vi "Retrieve and Convert Data.vi"(8 "error in (no error)":errorcluster, 11 "Variant In":variant) -> (0 "error out":errorcluster, 2 "Info":T1, 3 "Variant Out":variant)   [LabVIEW 2019, in "Inset.lvclass"]
uses:
  Inset.lvclass
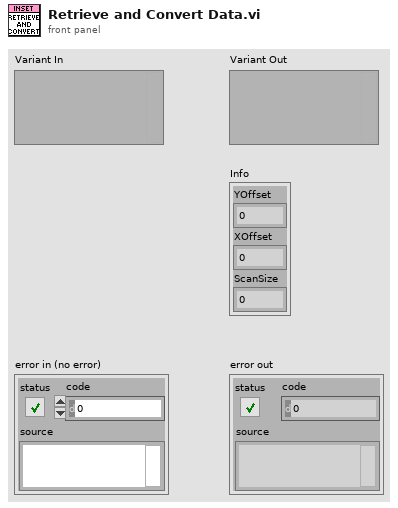
[diagram p1: front panel]
types:
  T1 = cluster{"YOffset":dbl, "XOffset":dbl, "ScanSize":dbl}
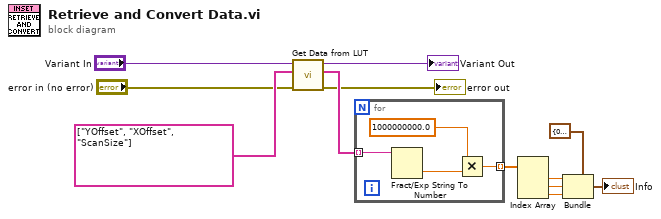
[diagram p0: block diagram]
diagram:
  n1 = call "Get Data from LUT.vi"("error in"="error in (no error)", "Keys"=string[] ["YOffset", "XOffset", "ScanSize"], "Variant In"="Variant In") -> ("error out"=→"error out":errorcluster, "Values"=w5:string[], "Variant Out"=→"Variant Out":variant)  [unwired: 6 in]
  n2 = for {
    tunnel: w5 -> [w16] mode=indexing
    tunnel: [w14] -> w12 mode=indexing
    n3 = Fract/Exp String To Number(string=w16) -> (number=w15:dbl)  [unwired: 3 in, 1 out]
    n4 = Multiply(x=1000000000.0, y=w15) -> (x*y=w14:dbl)
  }
  n5 = Index Array(array=w12) -> (element #1=w10:dbl, element #2=w9:dbl, element #3=w8:dbl)  [unwired: 3 in]
  n6 = Bundle(cluster=T1 {"YOffset"=0.0, "XOffset"=0.0, "ScanSize"=0.0}, "YOffset"=w10, "XOffset"=w9, "ScanSize"=w8) -> (→"Info":T1)
